vi "SplitterRefToSplitterIndexandElements.vi"(8 "error in (no error)":errorcluster, 10 "SplitterRef":refnum<vi>, 11 "PentaPanesGUI in":refnum<class "PentaPanes.lvclass">) -> (0 "error out":errorcluster, 1 "Splitter String":string, 2 "Splitter Pane Pos":T1 items=["Top", "Left", "Center", "Right", "Bottom"], 3 "PentaPanesGUI out":refnum<class "PentaPanes.lvclass">, 4 "Pressed Splitter Index Out":i32, 5 "Pane Ref out":refnum<vi>)   [LabVIEW 2022 SP3, in "PentaPanesLibrary.lvlib" / "PentaPanes.lvclass"]
uses:
  PentaPanes.lvclass
  PanePosition.ctl
  PentaPanes.lvclass/PentaPanes.ctl
  Read Top_Left_Right_Bottom arrays.vi
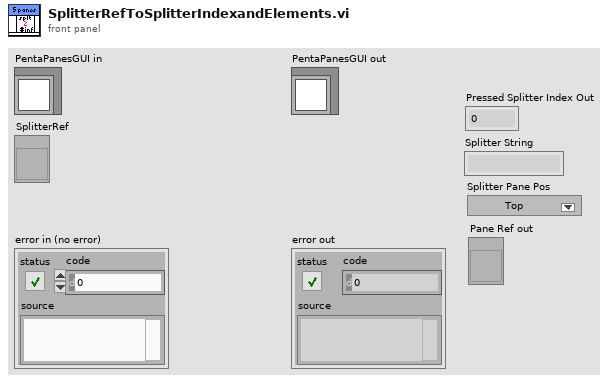
[diagram p1: front panel]
types:
  T1 = typedef "PentaPanesLibrary.lvlib/PentaPanes.lvclass/PanePosition.ctl" = u16
  T2 = typedef "PentaPanesLibrary.lvlib/PentaPanes.lvclass/TopLeftRightBottomArrays.ctl" = cluster{"Position Integer":T1[], "Position String":string[], "Splitter ref":refnum<vi>[], "Pane ref":refnum<vi>[]}
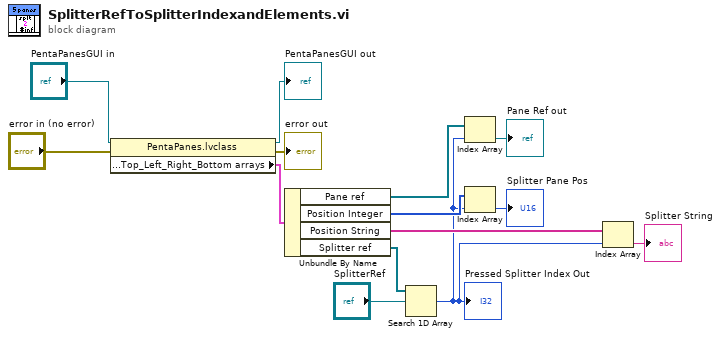
[diagram p0: block diagram]
diagram:
  n1 = property on="Property Node" class="PentaPanes.lvclass"(reference="PentaPanesGUI in", error in="error in (no error)") -> (reference out=→"PentaPanesGUI out":refnum<class "PentaPanes.lvclass">, error out=→"error out":errorcluster, "Public Methods:Helpers:Top_Left_Right_Bottom arrays"=w5:T2)
  n2 = Unbundle By Name(w5) -> ("Pane ref"=w11:refnum<vi>[], "Position Integer"=w6:T1[], "Position String"=w7:string[], "Splitter ref"=w8:refnum<vi>[])
  n3 = Search 1D Array(1D array=w8, element="SplitterRef") -> (index of element=w3:i32)  [unwired: 1 in]
  "Pressed Splitter Index Out" <- w3
  n4 = Index Array(array=w11, index=w3) -> (element=→"Pane Ref out":refnum<vi>)
  n5 = Index Array(array=w6, index=w3) -> (element=→"Splitter Pane Pos":T1)
  n6 = Index Array(array=w7, index=w3) -> (element=→"Splitter String":string)
